vi "Dashboard Main.vi"() -> ()   [LabVIEW 2013]
uses:
  <vilib>/event_ctls.llb/eventvkey.ctl
  <vilib>/Rock Robotics/WPI/Dashboard/WPI_DashboardLogging Global.vi
  <vilib>/Utility/config.llb/Write Key (String).vi
  <vilib>/Utility/config.llb/Write Key (I32).vi
  KariFramework/CheckImageDistance.vi
  <vilib>/Utility/config.llb/NI_LVConfig.lvlib
panel:
  in  "Enable Vision":bool=TRUE
  out "Image Message":string="Timeout in Camera Communications"
  in  "Rec Mode":enum32{"Stop", "Record", "Playback"}(radio)
  in  "Dashboard Tab":T1(tab)=enum."Auto"
  out "Gear":bool
  in  "AccelRate":dbl=2.5
  out "Distance":dbl
  out "RPM":dbl
  out "Error":bool
  out "Right Motor":dbl(slide) scale=-1.0..1.0 scale format="%#.6g"
  out "StraightDrive":bool
  out "HalfDrive":bool
  out "Left Motor":dbl(slide) scale=-1.0..1.0
  in  "Camera Settings":T2={"Frame Rate"=30, "Compression"=30, "Size"=1} {"Frame Rate" scale=1.0..30.0; "Size" items=["640x480", "320x240", "160x120"]}
  out "MotorSliders R":cluster{"MotorSlide1":dbl, "MotorSlide2":dbl} {"MotorSlide2" scale=-1.0..1.0 scale format="%#_2e"; "MotorSlide1" scale=-1.0..1.0 scale format="%#_2e"}
  out "MotorChart R":cluster{"Numeric":dbl, "Numeric":dbl}(graph)
  out "MotorSliders L":T3 {"MotorSlide4 2" scale=0.0..14.0 scale format="%#_2e"; "MotorSlide2" scale=-1.0..1.0 scale format="%#_2e"; "MotorSlide1" scale=-1.0..1.0 scale format="%#_2e"}
  out "MotorChart L":T4(graph)
  out "Mode":T5(ring)=enum."Auto Disabled"
  out "Camera IP":string
  in  "DB Camera Config":bool
  out "fps":dbl format="%#.1g"
  out "Mbps":dbl format="%#.1g"
  out "Mbps 2":bool
  in  "DesiredAngle":dbl step=11.25
  out "Angle":dbl
  in  "AccelScale":dbl=1.0 step=1.0
  in  "% Cutoff":dbl=0.5
  out "NumHot":i32
  out "NumProcessed":i32
  in  "NumSamples":i32=5
  out "ProcessImage?":bool
  in  "Finished?":bool
  in  "Hot?":bool
  in  "Score cutoff":dbl=0.5
  in  "Color System":u16(ring)=2 items=["RGB", "HSL", "HSV", "HSI"]
  out "Distance (ft)":dbl
  in  "Color Components":T6={"Hue"={112.0, 144.0}, "Sat"={202.0, 255.0}, "Val"={237.0, 255.0}} {"Val" scale=0.0..255.0; "Sat" scale=0.0..255.0; "Hue" scale=0.0..255.0 scale format="%#_3g"}
  out "LoopTime":u32
  in  "Reset?":bool
  in  "Test Slider":dbl(slide) scale=0.0..100.0 scale format="%#_3g"
  in  "On/Off":bool caption="Solenoid"
  in  "Test Name":u16(ring) items=["Select the test to run...", "Example Test", "-------------------------------", "List of tests is built in robot code.", "Replace with your own automated tests."]
  in  "Test Tree":string(tree)
  in  "Motor":cluster{"Value":dbl, "Enable":bool} {"Value" scale=-1.0..1.0 scale format="%#_3g"}
  out "Progress":T7 {"Test Progress" scale=0.0..100.0}
  in  "Rev/Fwd":cluster{"Forward":bool, "Reverse":bool}
  in  "Test Ring":u16(ring) items=["Auto", "Fixed indoor", "Fixed outdoor 1", "Fixed outdoor 2", "Fixed fluorescent 1", "Fixed fluorescent 2", "Hold current"]
  in  "Listbox":i32(listbox)
  out "Tree":string(tree)
  out "Errors":T8(array[cluster])
  in  "Reset":bool
  out "Camera Image":T9(plugin-control)
  # "Left"
  # "Front"
  # "Right"
  # "Battery"
  # "Customize by placing controls and indicators here and name to\nmatch Dashboard Variables on robot."
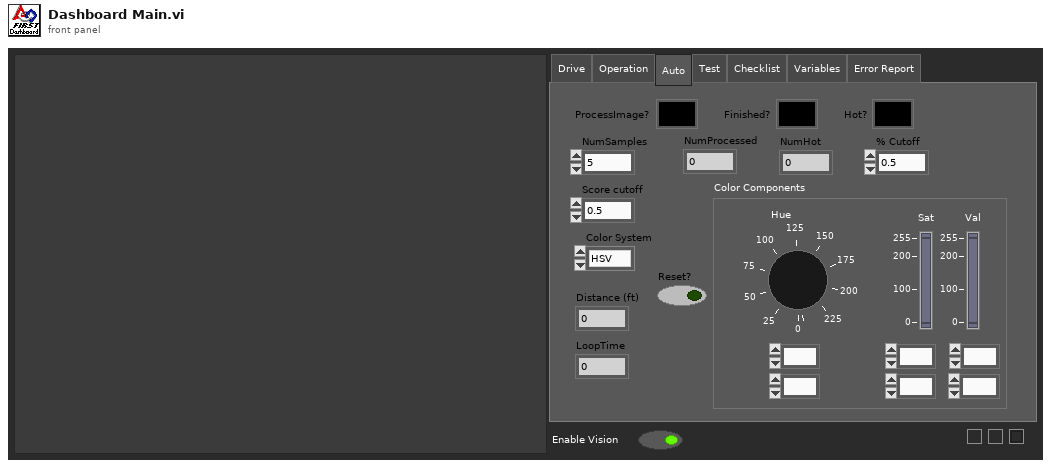
[diagram p1: front panel]
types:
  T1 = enum32{"Drive", "Operation", "Auto", "Test", "Checklist", "Variables", "Error Report"}
  T2 = cluster{"Frame Rate":i32, "Compression":i32, "Size":u16}
  T3 = cluster{"MotorSlide1":dbl, "MotorSlide2":dbl, "MotorSlide4 2":dbl}
  T4 = cluster{"Numeric":dbl, "Numeric":dbl, "Battery":sgl}
  T5 = enum8{"Tele-Op Disabled", "Tele-Op Enabled", "Auto Disabled", "Auto Enabled", "Test Disabled", "Test Enabled", ""}
  T6 = cluster{"Hue":cluster{dbl, dbl}, "Sat":cluster{dbl, dbl}, "Val":cluster{dbl, dbl}}
  T7 = cluster{"Test Progress":u8, "Test Progress Text":string}
  T8 = cluster{"status":bool, "code":i32, "location":string, "source":string}[]
  T9 = typedef "IMAQ Image.ctl" = refnum<image>
  T10 = enum32{"Drive", "Operation", "Auto", "Test", "Checklist", "Variables"}
  T11 = typedef "Image Type" = u32
  T12 = cluster{"Digital Inputs":bool[], "Digital Outputs":bool[]}
  T13 = cluster{"Competition mode":bool, "Robot Link":bool, "Autonomous":bool, "Enabled":bool, "E-Stop":bool, "Simulated":bool, "TestMode":bool, "Docked Window":bool}
  T14 = cluster{"Boolean":bool, "Numeric":i32, "String":string, "String":string}[]
  T15 = typedef "NI_LVConfig.lvlib/Config Data RefNum.ctl" = refnum<k1>
  T16 = typedef "eventvkey.ctl" = enum16{"ASCII", "Enter", "Return", "Shift", "Ctrl", "Alt", "Cmd", "Opt", "Caps", "NumLock", "Clear", "Break", "Up", "Down", "Left", "Right", "Insert", "Delete", "Home", "End", "PageUp", "PageDown", "Escape", "Help", "Pause", "ScrollLock", "F1", "F2", "F3", "F4", "F5", "F6", "F7", "F8", "F9", "F10", "F11", "F12", "F13", "F14", "F15", "F16", "F17", "F18", "F19", "F20", "F21", "F22", "F23", "F24", "Play", "VolumeUp", "VolumeDown", "Mute", "Two Byte Char"}
  T17 = cluster{"Image Size":bool, "Image Type":bool, "Pixel Value":bool, "ROI Information":bool, "Zoom Factor":bool}
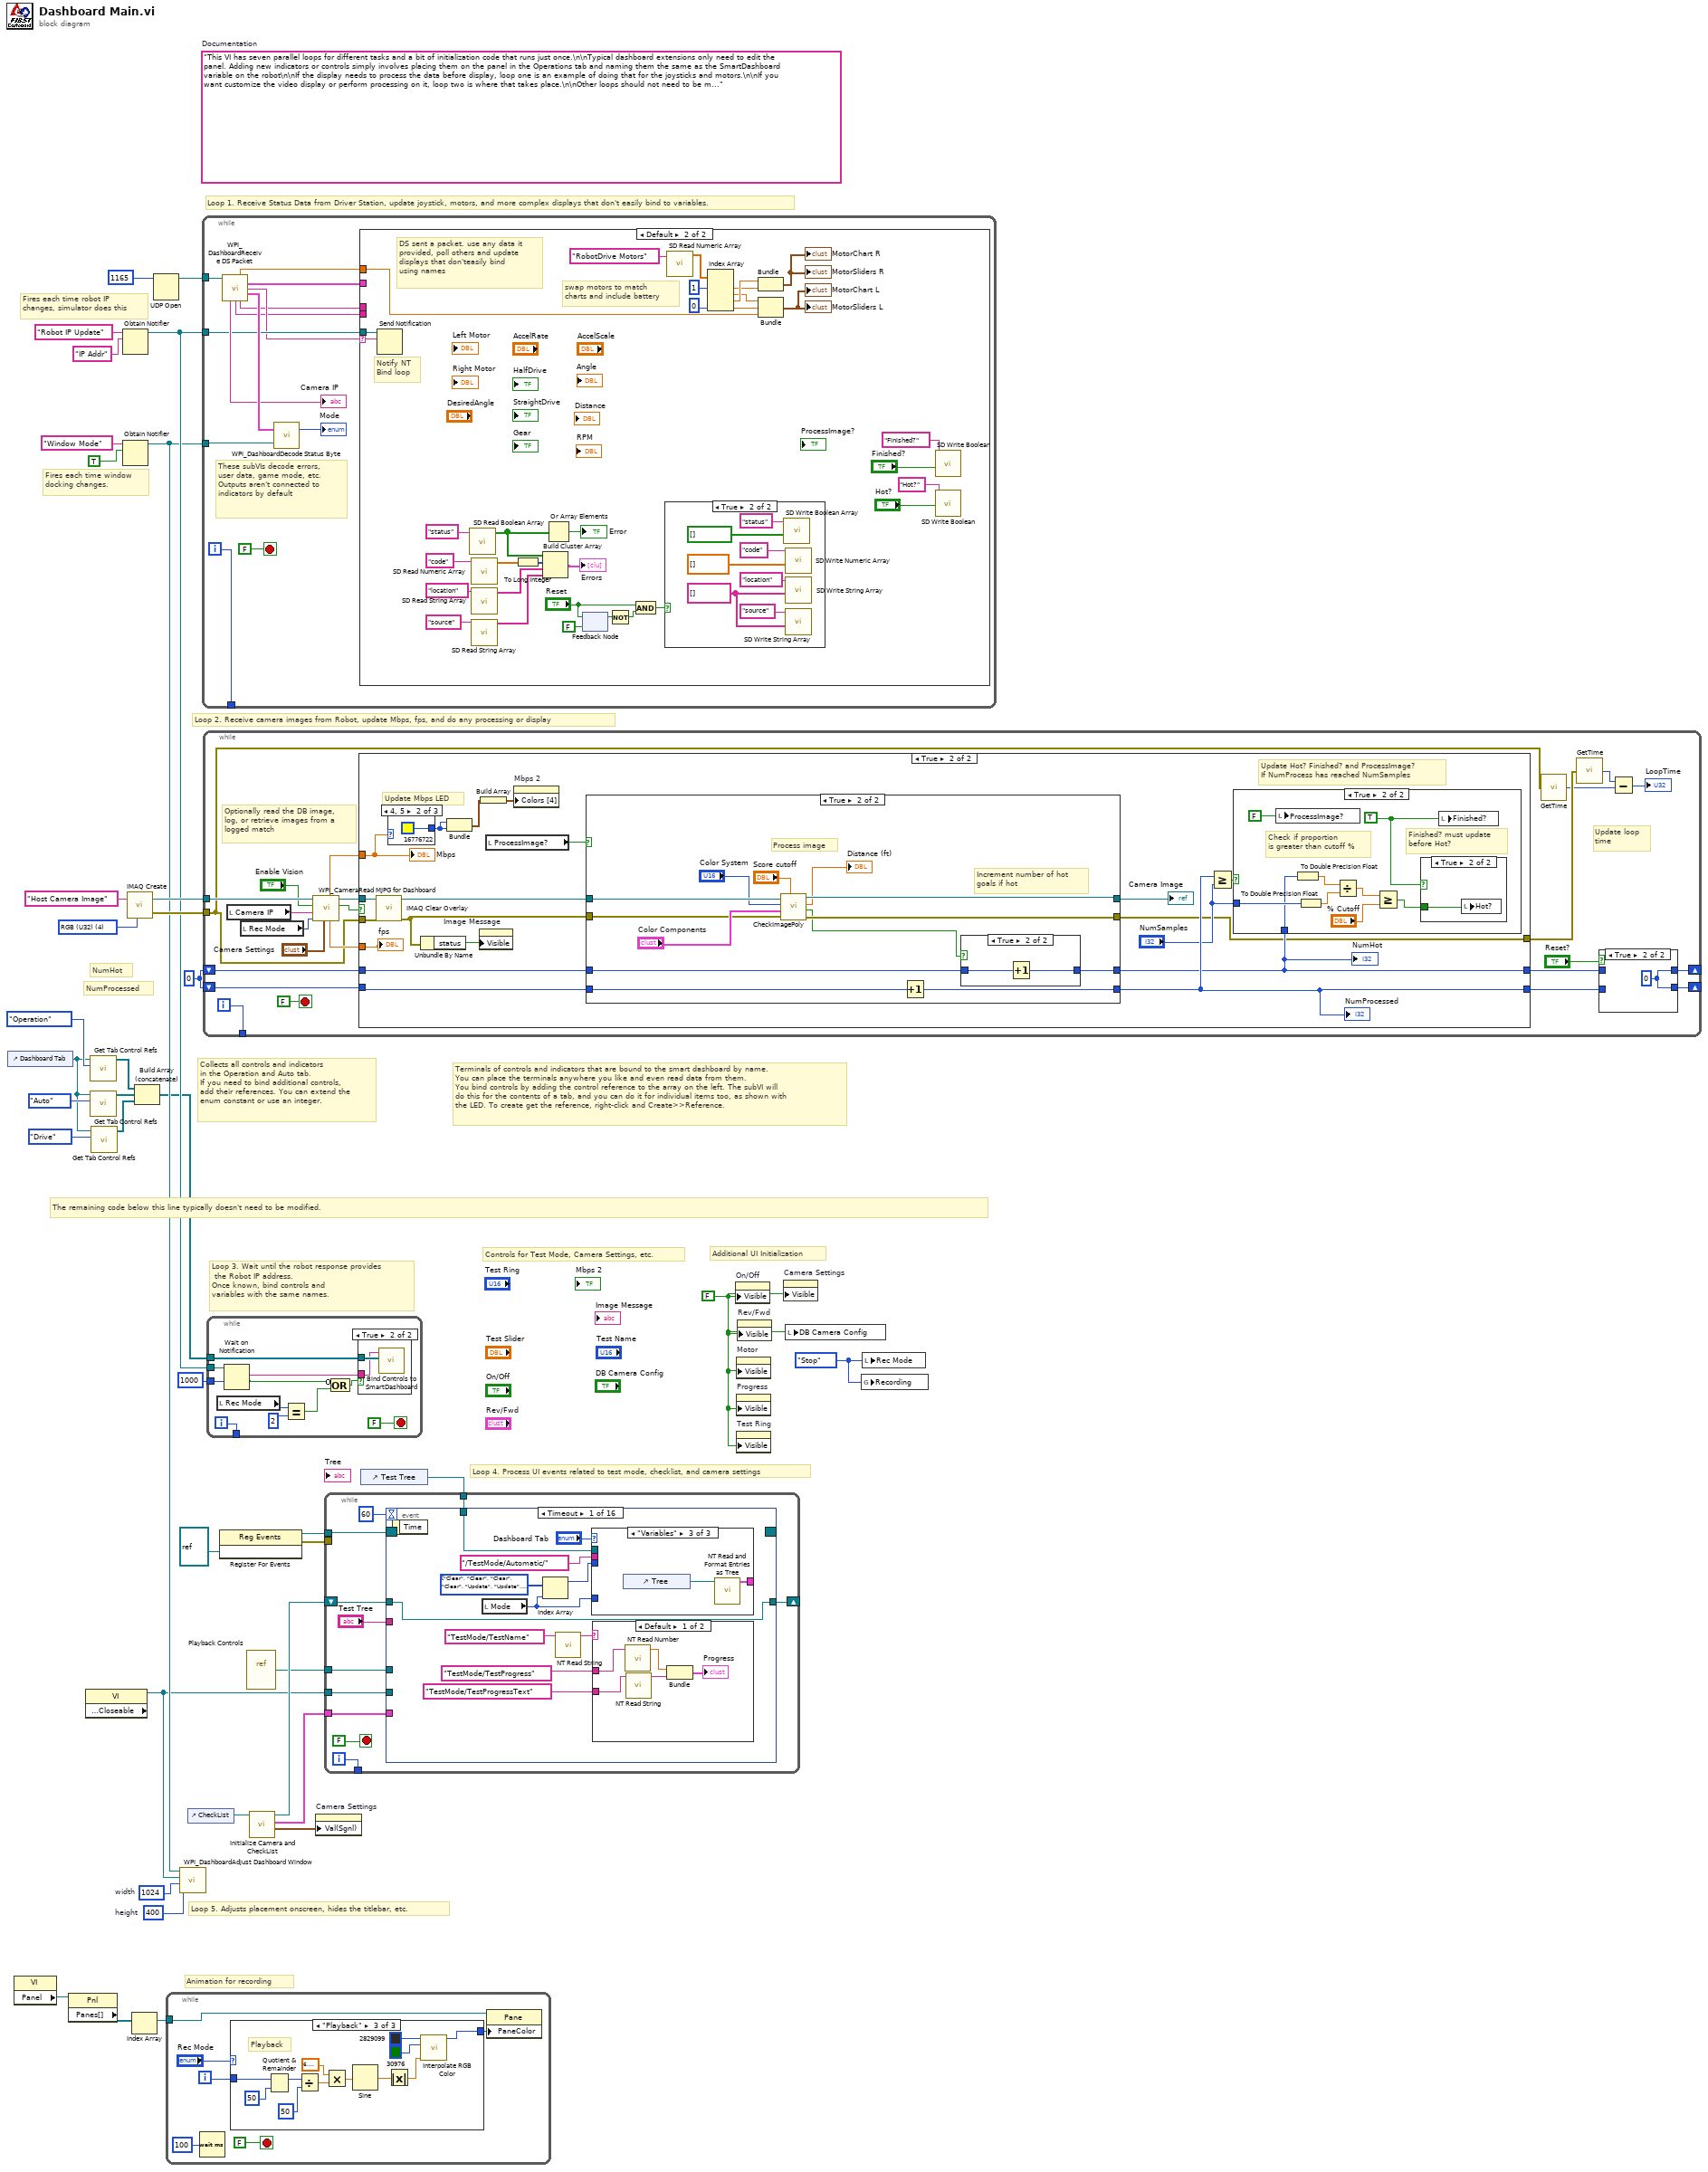
[diagram p0: block diagram]
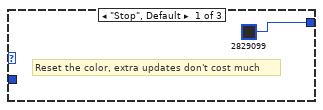
[diagram p2: hidden frame]
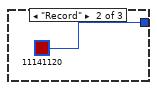
[diagram p3: hidden frame]
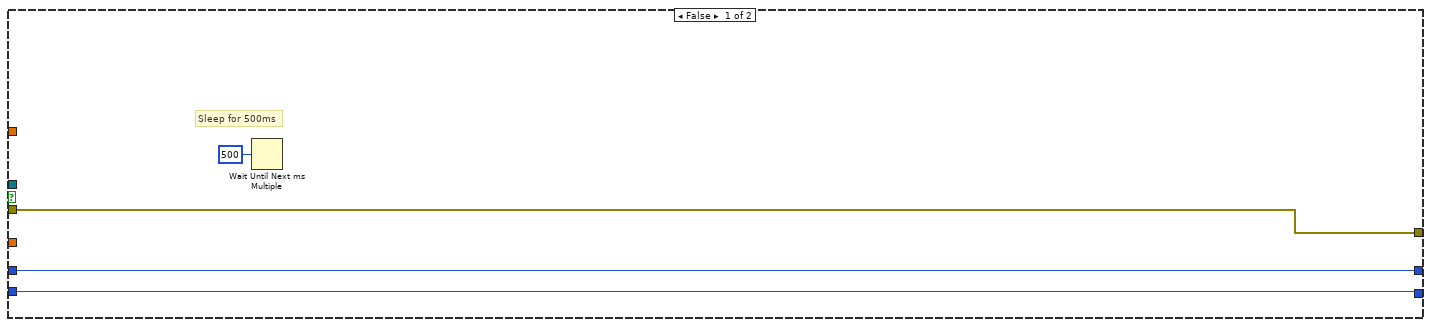
[diagram p6: hidden frame]
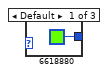
[diagram p11: hidden frame]
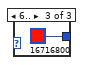
[diagram p12: hidden frame]
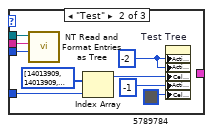
[diagram p14: hidden frame]
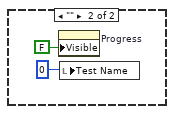
[diagram p15: hidden frame]
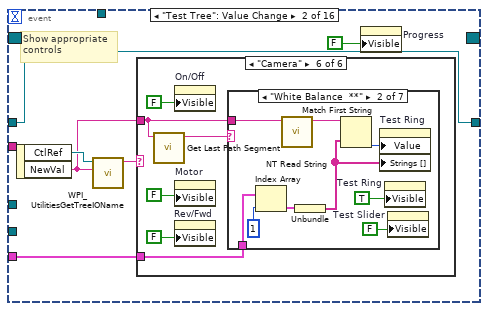
[diagram p16: hidden frame]
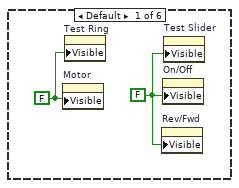
[diagram p17: hidden frame]
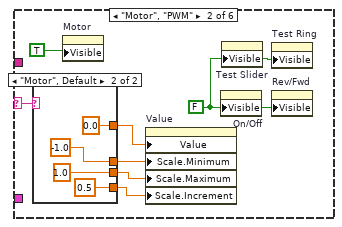
[diagram p18: hidden frame]
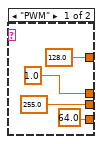
[diagram p19: hidden frame]
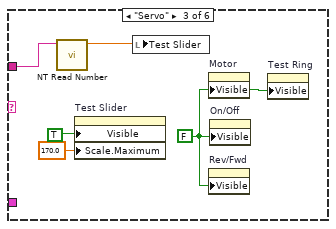
[diagram p20: hidden frame]
diagram:
  w1 = 0
  w10 = enum32{"Stop", "Record", "Playback"}."Stop" ("Rec Mode")
  w13 = 400  # height
  w14 = 1024  # width
  w27 = FALSE ("Visible")
  (unwired) "This VI has seven parallel loops for different tasks and a bit of initialization code that runs just once.\n\nTypical dashboard extensions only need to edit the panel. Adding new indicators or controls simply involves placing them on the panel in the Operations tab and naming them the same as the SmartDashboard variable on the robot\n\nIf the display needs to process the data before display, loop one is an example of doing that for the joysticks and motors.\n\nIf you want customize the video display or perform processing on it, loop two is where that takes place.\n\nOther loops should not need to be modified. They are pretty standard, and document the task they perform."  # Documentation
  w37 = T11 4 items=["Grayscale (U8)", "Grayscale (I16)", "Grayscale (SGL)", "Complex (CSG)", "RGB (U32)", "HSL (U32)", "RGB (U64)"] ("Image Type")
  # "NumProcessed"
  # "NumHot"
  # "Controls for Test Mode, Camera Settings, etc."
  # "Additional UI Initialization"
  # "Animation for recording"
  # "Fires each time robot IP\nchanges, simulator does this"
  # "Fires each time window\ndocking changes."
  # "Collects all controls and indicators\nin the Operation and Auto tab.\nIf you need to bind additional controls,\nadd their references. You can extend the\nenum constant or use an integer."
  # "The remaining code below this line typically doesn't need to be modified."
  # "Loop 4. Process UI events related to test mode, checklist, and camera settings"
  # "Terminals of controls and indicators that are bound to the smart dashboard by name.\nYou can place the terminals anywhere you like and even read data from them.\nYou bind controls by adding the control reference to the array on the left. The subVI will\ndo this for the contents of a tab, and you can do it for individual items too, as shown with\nthe LED. To create get the reference, right-click and Create>>Reference."
  # "Loop 3. Wait until the robot response provides\n the Robot IP address.\nOnce known, bind controls and\nvariables with the same names."
  # "Loop 5. Adjusts placement onscreen, hides the titlebar, etc."
  # "Loop 1. Receive Status Data from Driver Station, update joystick, motors, and more complex displays that don't easily bind to variables."
  # "Loop 2. Receive camera images from Robot, update Mbps, fps, and do any processing or display"
  n1 = control-ref of="Dashboard Tab"() -> (w3:refnum<vi>)
  n2 = property class="VI"() -> ("Panel"=w21:refnum<vi>)  [unwired: 2 in, 2 out]
  n3 = property class="Pnl"(reference=w21) -> ("Panes[]"=w22:refnum<vi>[])  [unwired: 1 in, 2 out]
  n4 = property class="VI" props=["Front Panel.Closeable"]() -> (reference out=w9:refnum<vi>)  [unwired: 2 in, 2 out]
  n5 = call <vilib>:"Get Tab Control Refs.vi"("Page Index"=T10."Operation" ("Dashboard Tab"), "TabControl in"=w3) -> ("ControlsOnPage"=w7:refnum<vi>[])  [unwired: 9 in]
  n6 = call <vilib>:"Get Tab Control Refs.vi"("Page Index"=T10."Auto" ("Dashboard Tab"), "TabControl in"=w3) -> ("ControlsOnPage"=w8:refnum<vi>[])  [unwired: 9 in]
  n7 = call <vilib>:"Get Tab Control Refs.vi"("Page Index"=T10."Drive" ("Dashboard Tab"), "TabControl in"=w3) -> ("ControlsOnPage"=w2:refnum<vi>[])  [unwired: 9 in]
  n8 = Obtain Notifier(name (unnamed)="Robot IP Update", notification data type="IP Addr" ("name (unnamed)")) -> (notifier out=w31:refnum<notifier>)  [unwired: 2 in, 2 out]
  n9 = Obtain Notifier(name (unnamed)="Window Mode", notification data type=TRUE) -> (notifier out=w12:refnum<notifier>)  [unwired: 2 in, 2 out]
  n10 = call "IMAQ Create"("Image Name"="Host Camera Image", "Image Type"=w37) -> ("New Image"=w35:T9, "error out"=w34:errorcluster)  [unwired: 2 in, 1 out]
  n11 = Index Array(array=w22) -> (element=w20:refnum<vi>)  [unwired: 1 in]
  n12 = Build Array (concatenate)(w7, w8, w2) -> (w6:refnum<vi>[])
  n13 = UDP Open(11:u16 1165 ("port")) -> (port=w38:refnum<k16>)  [unwired: 2 in, 4 out]
  n14 = while {
    tunnel: w20 -> [w41]
    i -> [w44]
    stop <- FALSE stop-if-true
    n15 = Wait (ms)(milliseconds to wait=u32 100) -> ()  [unwired: 1 out]
    n16 = case shown="\"Playback\"" "Rec Mode" {
      tunnel: w44 -> [_ _ w59]
      tunnel: [u32 2829099 ("Base Color") u32 11141120 ("Target Color") w48] -> w40
      frame "Stop", Default {
        # "Reset the color, extra updates don't cost much"
      }
      frame "Record" {
      }
      frame "Playback" {
        # "Playback"
        n17 = Quotient & Remainder(x=w59, y=u32 50 ("milliseconds to wait")) -> (x-y*floor(x/y)=w55:u32)  [unwired: 1 out]
        n18 = Divide(x=w55, y=u32 50 ("milliseconds to wait")) -> (x/y=w52:dbl)
        n19 = Multiply(x=6.283185307179586, y=w52) -> (x*y=w57:dbl)
        n20 = Sine(x=w57) -> (sin(x)=w56:dbl)
        n21 = Absolute Value(x=w56) -> (abs(x)=w49:dbl)
        n22 = call "Interpolate RGB Color.vi"("Proportion"=w49, "Target Color"=u32 30976, "Base Color"=u32 2829099) -> ("Result Color"=w48:u32)  [unwired: 8 in]
      }
    }
    n23 = property class="Pane"(reference=w41, "PaneColor"=w40) -> ()  [unwired: 1 in, 2 out]
  }
  n24 = call <vilib>:"WPI_DashboardAdjust Dashboard Window.vi"("height"=w13, "width"=w14, "reference in"=w9, "Notifier in"=w12) -> ()  [unwired: 8 in]
  n25 = control-ref of="CheckList"() -> (w11:refnum<vi>)
  n26 = while {
    tunnel: w38 -> [w70]
    tunnel: w31 -> [w65]
    tunnel: w12 -> [w69]
    tunnel: [w66] -> _
    i -> [w66]
    stop <- FALSE stop-if-true
    # "These subVIs decode errors, user data, game mode, etc.\nOutputs aren't connected to indicators by default"
    n27 = call <vilib>:"WPI_DashboardReceive DS Packet.vi"("Recv Socket"=w70) -> ("Battery"=w60:sgl, "Driver Station"=w61:T12, "Robot IP Address"=w64:string, "Status"=w71:T13, "Camera IP Address"=→"Camera IP":string, "Low Priority User Data"=w63:string, "High Priority User Data"=w62:string)  [unwired: 1 in, 7 out]
    n28 = call <vilib>:"WPI_DashboardDecode Status Byte.vi"("Window Mode Notifier"=w69, "Status"=w71) -> ("Mode"=→"Mode":T5)  [unwired: 1 out]
    n29 = case shown="Default" w64 {
      selector: w64 -> [_ w103]
      tunnel: w65 -> [_ w104]
      tunnel: w63 -> [_ _]
      tunnel: w62 -> [_ _]
      tunnel: w61 -> [_ _]
      tunnel: w60 -> [_ w102]
      frame "0.0.0.0" {
        # "DS not sending packets, or no robot exists yet.\nDon't poll the variables"
      }
      frame Default {
        # "Notify NT\nBind loop"
        # "DS sent a packet. use any data it\nprovided, poll others and update\ndisplays that don'teasily bind\nusing names"
        # "swap motors to match\ncharts and include battery"
        n30 = Send Notification(notification=w103, notifier=w104) -> ()  [unwired: 1 in, 2 out]
        n31 = call <vilib>:"SD Read Boolean Array.vi"("Name"="status") -> ("Boolean Array"=w82:bool[])  [unwired: 8 in, 2 out]
        n32 = call <vilib>:"SD Read Numeric Array.vi"("Name"="code") -> ("Numeric Array"=w81:dbl[])  [unwired: 8 in, 2 out]
        n33 = call <vilib>:"SD Read String Array.vi"("Name"="location") -> ("String Array"=w80:string[])  [unwired: 9 in, 1 out]
        n34 = call <vilib>:"SD Read String Array.vi"("Name"="source") -> ("String Array"=w79:string[])  [unwired: 9 in, 1 out]
        n35 = To Long Integer(number=w81) -> (32bit integer=w87:i32[])
        n36 = Build Cluster Array(w82, w87, w80, w79) -> (→"Errors":T14)
        n37 = Or Array Elements(Boolean array=w82) -> (logical OR=→"Error":bool)
        n38 = feedback #1(FALSE ("Reset")) -> (w90:bool)
        n39 = feedback-in #1("Reset") -> ()
        n40 = Not(x=w90) -> (.not. x?=w89:bool)
        n41 = And(x="Reset", y=w89) -> (x .and. y?=w88:bool)
        n42 = case shown="True" w88 {
          frame False {
          }
          frame True {
            w106 = string[] [] ("String Array")
            n43 = call <vilib>:"SD Write Boolean Array.vi"("Boolean Array"=bool[] [], "Name"="status") -> ()  [unwired: 8 in, 2 out]
            n44 = call <vilib>:"SD Write Numeric Array.vi"("Numeric Array"=dbl[] [], "Name"="code") -> ()  [unwired: 8 in, 2 out]
            n45 = call <vilib>:"SD Write String Array.vi"("String Array"=w106, "Name"="location") -> ()  [unwired: 8 in, 2 out]
            n46 = call <vilib>:"SD Write String Array.vi"("String Array"=w106, "Name"="source") -> ()  [unwired: 8 in, 2 out]
          }
        }
        n47 = call <vilib>:"SD Read Numeric Array.vi"("Name"="RobotDrive Motors") -> ("Numeric Array"=w101:dbl[])  [unwired: 8 in, 2 out]
        n48 = Index Array(array=w101, index #1=1, index #4=0) -> (element #1=w97:dbl, element #2=w96:dbl, element #3=w98:dbl, element #4=w93:dbl)  [unwired: 2 in]
        n49 = Bundle("Numeric"=w98, "Numeric"=w97) -> (→"MotorChart R" →"MotorSliders R":cluster{"Numeric":dbl, "Numeric":dbl})  [unwired: 1 in]
        n50 = Bundle("Numeric"=w96, "Numeric"=w93, "Battery"=w102) -> (→"MotorChart L" →"MotorSliders L":T4)  [unwired: 1 in]
        n51 = call <vilib>:"SD Write Boolean.vi"("Boolean"="Finished?", "Name"="Finished?") -> ()  [unwired: 8 in, 2 out]
        n52 = call <vilib>:"SD Write Boolean.vi"("Boolean"="Hot?", "Name"="Hot?") -> ()  [unwired: 8 in, 2 out]
      }
    }
  }
  n53 = while {
    tunnel: w35 -> [w133]
    tunnel: w34 -> [w118]
    tunnel: [w134] -> _
    shift-right: [w115] -> _
    shift-left: w1 -> [w123]
    shift-right: [w116] -> _
    shift-left: w1 -> [w124]
    i -> [w134]
    stop <- FALSE stop-if-true
    # "Update loop\ntime"
    # "Optionally read the DB image,\nlog, or retrieve images from a\nlogged match"
    n54 = local read "Camera IP"() -> (w126:string)
    n55 = local read "Rec Mode"() -> (w125:enum32{"Stop", "Record", "Playback"})
    n56 = call <vilib>:"WPI_CameraRead MJPG for Dashboard.vi"("Camera Settings"="Camera Settings", "Rec Mode"=w125, "Camera IP"=w126, "Enable"="Enable Vision", "Refnum in"=w133) -> ("Active"=w130:bool, "Refnum out"=w132:T9, "FPS"=w129:dbl, "Bandwidth (Mbps)"=w128:dbl)  [unwired: 3 in]
    n57 = case shown="True" w130 {
      tunnel: w132 -> [_ w157]
      tunnel: w128 -> [_ w156]
      tunnel: w129 -> [_ w155]
      tunnel: w124 -> [w140 w152]
      tunnel: w123 -> [w141 w151]
      tunnel: [w141 w148] -> w113
      tunnel: [w140 w147] -> w114
      tunnel: [w139 w145] -> w121
      tunnel: w118 -> [w139 w144]
      frame False {
        # "Sleep for 500ms"
        n58 = Wait Until Next ms Multiple(millisecond multiple=u32 500) -> ()  [unwired: 1 out]
      }
      frame True {
        # "Update Hot? Finished? and ProcessImage?\nIf NumProcess has reached NumSamples"
        # "Update Mbps LED"
        n59 = call "IMAQ Clear Overlay"("error in (no error)"=w144, "Image"=w157) -> ("error out"=w150:errorcluster, "Image Out"=w154:T9)  [unwired: 1 in, 7 out]
        n60 = case shown="4, 5" w156 {
          tunnel: [u32 6618880 ("Color Box") u32 16776722 ("Color Box") u32 16716800 ("Color Box")] -> w158
          frame Default {
          }
          frame 4, 5 {
          }
          frame 6.. {
          }
        }
        n61 = Unbundle By Name(w150) -> ("status"=w161:bool)
        n62 = Bundle("Color Box"=w158, "Color Box"=w158) -> (w160:cluster{"Color Box":u32, "Color Box":u32})  [unwired: 1 out]
        n63 = property on="Image Message" class="Str"("Visible"=w161) -> ()  [unwired: 2 in, 2 out]
        n64 = Build Array(w160) -> (w159:cluster{"Color Box":u32, "Color Box":u32}[])
        n65 = local read "ProcessImage?"() -> (w143:bool)
        n66 = property on="Mbps 2" class="Bool (strict)"("Colors [4]"=w159) -> ()  [unwired: 2 in, 2 out]
        n67 = case shown="True" w143 {
          tunnel: w154 -> [w175 w188]
          tunnel: [w175 w182] -> w153
          tunnel: w152 -> [w173 w179]
          tunnel: w151 -> [w174 w181]
          tunnel: w150 -> [w172 w184]
          tunnel: [w172 w183] -> w145
          tunnel: [w174 w180] -> w148
          tunnel: [w173 w178] -> w147
          frame False {
          }
          frame True {
            # "Process image"
            # "Increment number of hot\ngoals if hot"
            n68 = call-poly "CheckImagePoly.vi"("Score cutoff"="Score cutoff", "error in"=w184, "Color Components"="Color Components", "Color System"="Color System", "Image"=w188) -> ("error out"=w183:errorcluster, "Hot?"=w176:bool, "Distance (ft)"=→"Distance (ft)":dbl, "Image out"=w182:T9)  [unwired: 3 in]
            n69 = Increment(x=w181) -> (x+1=w180:i32)
            n70 = case shown="True" w176 {
              tunnel: w179 -> [w189 w191]
              tunnel: [w189 w190] -> w178
              frame False {
              }
              frame True {
                n71 = Increment(x=w191) -> (x+1=w190:i32)
              }
            }
          }
        }
        "Camera Image" <- w153
        "NumHot" <- w147
        "NumProcessed" <- w148
        n72 = Greater Or Equal?(x=w148, y="NumSamples") -> (x >= y?=w149:bool)
        n73 = case shown="True" w149 {
          tunnel: w147 -> [_ w169]
          tunnel: "NumSamples" -> [_ w170]
          frame False {
          }
          frame True {
            w162 = TRUE ("Finished?")
            # "Finished? must update\nbefore Hot?"
            # "Check if proportion\nis greater than cutoff %"
            n74 = local write "ProcessImage?"(FALSE ("ProcessImage?")) -> ()
            n75 = To Double Precision Float(number=w169) -> (double precision float=w167:dbl)
            n76 = To Double Precision Float(number=w170) -> (double precision float=w168:dbl)
            n77 = Divide(x=w167, y=w168) -> (x/y=w166:dbl)
            n78 = Greater Or Equal?(x=w166, y="% Cutoff") -> (x >= y?=w164:bool)
            n79 = case shown="True" w162 {
              tunnel: w164 -> [_ w171]
              frame False {
              }
              frame True {
                n80 = local write "Hot?"(w171) -> ()
              }
            }
            n81 = local write "Finished?"(w162) -> ()
          }
        }
        "Mbps" <- w156
        "fps" <- w155
      }
    }
    n82 = call "GetTime.vi"("error in"=w118) -> ("Time"=w120:u32)
    n83 = call "GetTime.vi"("error in"=w121) -> ("Time"=w122:u32)
    n84 = case shown="True" "Reset?" {
      tunnel: [w137 w138] -> w116
      tunnel: [w136 w138] -> w115
      tunnel: w114 -> [w137 _]
      tunnel: w113 -> [w136 _]
      frame False {
      }
      frame True {
        w138 = 0
      }
    }
    n85 = Subtract(x=w122, y=w120) -> (x-y=→"LoopTime":u32)
  }
  n86 = while {
    tunnel: w6 -> [w205]
    tunnel: w31 -> [w203]
    tunnel: [w201] -> _
    tunnel: u32 1000 ("milliseconds to wait") -> [w200]
    i -> [w201]
    stop <- FALSE stop-if-true
    n87 = local read "Rec Mode"() -> (w196:enum32{"Stop", "Record", "Playback"})
    n88 = Wait on Notification(notifier=w203, timeout in ms (-1)=w200) -> (notification=w202:string, timed out?=w198:bool)  [unwired: 2 in, 2 out]
    n89 = Equal?(x=w196, y=u16 2 ("Rec Mode")) -> (x = y?=w197:bool)
    n90 = Compound Arithmetic op=OR(invert w198, w197) -> (w199:bool)
    n91 = case shown="True" w199 {
      tunnel: w205 -> [_ w207]
      tunnel: w202 -> [_ w206]
      frame False {
      }
      frame True {
        n92 = call <vilib>:"Bind Controls to SmartDashboard.vi"("Bound Control Refs"=w207, "Server IP Address"=w206) -> ()  [unwired: 10 in]
      }
    }
  }
  n93 = register-events(refnum<vi> refnum) -> (reference out=w18:refnum<event-registration>, error out=w17:errorcluster)  [unwired: 2 in]
  n94 = vi-ref "Playback Controls.vi"() -> (w19:refnum<vi>)
  n95 = call "Initialize Camera and CheckList.vi"("ListBox in"=w11) -> ("Cluster"=w25:cluster{"value":i32, "value":i32, "index":i32}, "Array"=w26:cluster{string[]}[], "File Refnum"=w24:T15)  [unwired: 8 in]
  n96 = property on="Camera Settings" class="Clust (strict)"("Val(Sgnl)"=w25) -> ()  [unwired: 2 in, 2 out]
  n97 = control-ref of="Test Tree"() -> (w23:refnum<vi>)
  n98 = while {
    tunnel: w26 -> [w215]
    shift-right: [w214] -> _
    shift-left: w24 -> [w213]
    tunnel: [w212] -> _
    tunnel: w23 -> [w211]
    tunnel: w19 -> [w210]
    tunnel: w18 -> [w209]
    tunnel: w17 -> [_]
    tunnel: w9 -> [w208]
    i -> [w212]
    stop <- FALSE stop-if-true
    n99 = event shown="[0] Timeout" {
      selector: w209 -> [_ _ _ _ _ _ _ _ _ _ _ _ _ _ _ _]
      dyn-events: [_ _ _ _ _ _ _ _ _ _ _ _ _ w453 _ _] -> _
      timeout: u32 60 ("milliseconds to wait") -> [_ _ _ _ _ _ _ _ _ _ _ _ _ _ _ _]
      tunnel: w211 -> [w225 _ _ _ _ _ _ _ _ _ _ _ _ _ _ _]
      tunnel: "Test Tree" -> [_ _ _ _ _ _ _ _ w422 w430 w432 w436 w444 _ _ _]
      tunnel: w215 -> [_ w249 _ _ _ _ w386 w416 _ _ _ _ _ _ _ _]
      tunnel: [w219 w248 w347 w352 w360 w372 w385 w409 w421 w428 w431 w435 w443 w455 w469 w470] -> w214
      tunnel: w213 -> [w219 w248 w347 w352 w360 w372 w384 w409 w421 w428 w431 w435 w443 w455 w469 w470]
      tunnel: w210 -> [_ _ _ _ _ _ _ _ _ _ _ _ _ w456 _ w473]
      tunnel: w208 -> [_ _ _ _ _ _ _ _ _ _ _ _ _ w451 _ _]
      event Timeout {
        w224 = enum16{"Update", "Clear"}[] [enum."Clear", enum."Clear", enum."Clear", enum."Clear", enum."Update", enum."Update", enum."Clear"] items=["Update", "Clear"]
        n100 = event-data() -> ()  [unwired: 1 in, 1 out]
        n101 = local read "Mode"() -> (w222:T5)
        n102 = Index Array(array=w224, index=w222) -> (element=w223:enum16{"Update", "Clear"})
        n103 = call <vilib>:"NT Read String.vi"("Name"="TestMode/TestName") -> ("String"=w228:string)  [unwired: 9 in, 1 out]
        n104 = case shown="\"Variables\"" "Dashboard Tab" {
          tunnel: w225 -> [_ w238 _]
          tunnel: "/TestMode/Automatic/" ("Name Pattern") -> [_ w237 _]
          tunnel: w223 -> [_ w236 _]
          tunnel: w222 -> [_ w234 _]
          tunnel: [_ _ w240] -> _
          frame "Operation", Default {
          }
          frame "Test" {
            w233 = -2 ("Active Item:Row Number")
            n105 = call <vilib>:"NT Read and Format Entries as Tree.vi"("Operation"=w236, "Name Pattern"=w237, "Tree Refnum"=w238) -> ()  [unwired: 7 in, 2 out]
            n106 = Index Array(array=u32[] [14013909, 14013909, 14013909, 14013909, 14013909, 16777215, 14013909], index=w234) -> (element=w232:u32)
            n107 = property on="Test Tree" class="Tree (strict)"("Active Item Row Number"=w233, "ActiveColNum"=w233, "CellBG"=w232, "Active Item Row Number"=-1 ("Active Item:Row Number"), "CellBG"=u32 5789784 ("Color Box")) -> ()  [unwired: 2 in, 2 out]
          }
          frame "Variables" {
            n108 = control-ref of="Tree"() -> (w239:refnum<vi>)
            n109 = call <vilib>:"NT Read and Format Entries as Tree.vi"("Tree Refnum"=w239) -> ("Formatted Strings"=w240:cluster{"Name":string, "Value":string}[])  [unwired: 9 in, 1 out]
          }
        }
        n110 = case shown="Default" w228 {
          tunnel: "TestMode/TestProgress" ("Name") -> [w242 _]
          tunnel: "TestMode/TestProgressText" ("Name") -> [w241 _]
          frame Default {
            n111 = call <vilib>:"NT Read Number.vi"("Name"=w242) -> ("Numeric"=w243:dbl)  [unwired: 9 in, 1 out]
            n112 = call <vilib>:"NT Read String.vi"("Name"=w241) -> ("String"=w244:string)  [unwired: 9 in, 1 out]
            n113 = Bundle("Numeric"=w243, "String"=w244) -> (→"Progress":cluster{"Numeric":dbl, "String":string})  [unwired: 1 in]
          }
          frame "" {
            n114 = property on="Progress" class="Clust (strict)"("Visible"=FALSE) -> ()  [unwired: 2 in, 2 out]
            n115 = local write "Test Name"(u16 0) -> ()
          }
        }
      }
      event "Test Tree": Value Change {
        # "Show appropriate\ncontrols"
        n116 = event-data() -> ("CtlRef"=w252:refnum<vi>, "NewVal"=w250:string)  [unwired: 1 in]
        n117 = call <vilib>:"WPI_UtilitiesGetTreeIOName.vi"("NewVal"=w250, "TreeControl in"=w252) -> ("I/O Name"=w253:string)  [unwired: 9 in]
        n118 = case shown="\"Camera\"" w253 {
          selector: w253 -> [_ w260 _ w278 w287 _]
          tunnel: w250 -> [_ _ w275 w277 _ w294]
          tunnel: w249 -> [_ _ _ _ _ w293]
          frame Default {
            w255 = FALSE ("Visible")
            w254 = FALSE ("Visible")
            n119 = property on="Motor" class="Clust (strict)"("Visible"=w254) -> ()  [unwired: 2 in, 2 out]
            n120 = property on="Test Ring" class="Ring (strict)"("Visible"=w254) -> ()  [unwired: 2 in, 2 out]
            n121 = property on="Rev/Fwd" class="Clust (strict)"("Visible"=w255) -> ()  [unwired: 2 in, 2 out]
            n122 = property on="On/Off" class="Bool (strict)"("Visible"=w255) -> ()  [unwired: 2 in, 2 out]
            n123 = property on="Test Slider" class="Slide (strict)"("Visible"=w255) -> ()  [unwired: 2 in, 2 out]
          }
          frame "Motor", "PWM" {
            w261 = FALSE ("Visible")
            n124 = case shown="\"Motor\", Default" w260 {
              tunnel: [1.0 ("Value") -1.0 ("Value")] -> w259
              tunnel: [255.0 ("Value") 1.0 ("Value")] -> w258
              tunnel: [128.0 ("Value") 0.0 ("Value")] -> w257
              tunnel: [64.0 ("Value") 0.5 ("Value")] -> w256
              frame "PWM" {
              }
              frame "Motor", Default {
              }
            }
            n125 = property on="Motor" class="Clust (strict)"("Visible"=TRUE) -> ()  [unwired: 2 in, 2 out]
            n126 = property on="Value" class="Slide (strict)"("Value"=w257, "Scale.Minimum"=w259, "Scale.Maximum"=w258, "Scale.Increment"=w256) -> ()  [unwired: 2 in, 2 out]
            n127 = property on="On/Off" class="Bool (strict)"("Visible"=w261) -> ()  [unwired: 2 in, 2 out]
            n128 = property on="Test Slider" class="Slide (strict)"("Visible"=w261) -> ()  [unwired: 2 in, 2 out]
            n129 = property on="Test Ring" class="Ring (strict)"("Visible"=w261) -> ()  [unwired: 2 in, 2 out]
            n130 = property on="Rev/Fwd" class="Clust (strict)"("Visible"=w261) -> ()  [unwired: 2 in, 2 out]
          }
          frame "Servo" {
            w273 = FALSE ("Visible")
            n131 = call <vilib>:"NT Read Number.vi"("Name"=w275) -> ("Numeric"=w274:dbl)  [unwired: 9 in, 1 out]
            n132 = property on="Test Slider" class="Slide (strict)"("Visible"=TRUE, "Scale.Maximum"=170.0 ("Scale.Range:Maximum")) -> ()  [unwired: 2 in, 2 out]
            n133 = local write "Test Slider"(w274) -> ()
            n134 = property on="Motor" class="Clust (strict)"("Visible"=w273) -> ()  [unwired: 2 in, 2 out]
            n135 = property on="Rev/Fwd" class="Clust (strict)"("Visible"=w273) -> ()  [unwired: 2 in, 2 out]
            n136 = property on="On/Off" class="Bool (strict)"("Visible"=w273) -> ()  [unwired: 2 in, 2 out]
            n137 = property on="Test Ring" class="Ring (strict)"("Visible"=w273) -> ()  [unwired: 2 in, 2 out]
          }
          frame "Relay", "Solenoid" {
            w276 = FALSE ("Visible")
            n138 = property on="Motor" class="Clust (strict)"("Visible"=w276) -> ()  [unwired: 2 in, 2 out]
            n139 = property on="Test Slider" class="Slide (strict)"("Visible"=w276) -> ()  [unwired: 2 in, 2 out]
            n140 = Search and Replace String(input string=w277, search string="/Value  **", replace string="/Direction") -> (result string=w283:string)  [unwired: 5 in, 3 out]
            n141 = property on="Test Ring" class="Ring (strict)"("Visible"=w276) -> ()  [unwired: 2 in, 2 out]
            n142 = call <vilib>:"NT Read String.vi"("Name"=w283) -> ("String"=w281:string)  [unwired: 9 in, 1 out]
            n143 = Equal?(x="Both directions", y=w281) -> (x = y?=w279:bool)
            n144 = Not(x=w279) -> (.not. x?=w280:bool)
            n145 = property on="Rev/Fwd" class="Clust (strict)"("Visible"=w279) -> ()  [unwired: 2 in, 2 out]
            n146 = property on="On/Off" class="Bool (strict)"("Visible"=w280, "Caption.Text"=w278) -> ()  [unwired: 2 in, 2 out]
          }
          frame "Compressor", "Digital Out" {
            w286 = FALSE ("Visible")
            # "Get direction and finish"
            n147 = property on="Motor" class="Clust (strict)"("Visible"=w286) -> ()  [unwired: 2 in, 2 out]
            n148 = property on="Test Slider" class="Slide (strict)"("Visible"=w286) -> ()  [unwired: 2 in, 2 out]
            n149 = property on="Test Ring" class="Ring (strict)"("Visible"=w286) -> ()  [unwired: 2 in, 2 out]
            n150 = property on="On/Off" class="Bool (strict)"("Visible"=TRUE, "Caption.Text"=w287) -> ()  [unwired: 2 in, 2 out]
            n151 = property on="Rev/Fwd" class="Clust (strict)"("Visible"=FALSE) -> ()  [unwired: 2 in, 2 out]
          }
          frame "Camera" {
            n152 = call <vilib>:"Get Last Path Segment.vi"("String in"=w294) -> ("String out"=w295:string)  [unwired: 10 in]
            n153 = property on="On/Off" class="Bool (strict)"("Visible"=FALSE) -> ()  [unwired: 2 in, 2 out]
            n154 = property on="Motor" class="Clust (strict)"("Visible"=FALSE) -> ()  [unwired: 2 in, 2 out]
            n155 = property on="Rev/Fwd" class="Clust (strict)"("Visible"=FALSE) -> ()  [unwired: 2 in, 2 out]
            n156 = case shown="\"White Balance  **\"" w295 {
              tunnel: w294 -> [w301 w310 w319 w328 w337 _ w343]
              tunnel: w293 -> [w299 w307 w316 w325 w334 _ _]
              frame "Size  **" {
                n157 = Index Array(array=w299) -> (element=w298:cluster{string[]})  [unwired: 1 in]
                n158 = call <vilib>:"NT Read String.vi"("Name"=w301) -> ("String"=w300:string)  [unwired: 9 in, 1 out]
                n159 = Unbundle(w298) -> (w296:string[])
                n160 = Match First String(2:w296, 3:w300) -> (0:w297:i32)  [unwired: 1 out]
                n161 = property on="Test Ring" class="Ring (strict)"("Value"=w297, "Strings []"=w296) -> ()  [unwired: 2 in, 2 out]
                n162 = property on="Test Ring" class="Ring (strict)"("Visible"=TRUE) -> ()  [unwired: 2 in, 2 out]
                n163 = property on="Test Slider" class="Slide (strict)"("Visible"=FALSE) -> ()  [unwired: 2 in, 2 out]
              }
              frame "White Balance  **" {
                n164 = Index Array(array=w307, index=1) -> (element=w308:cluster{string[]})
                n165 = call <vilib>:"NT Read String.vi"("Name"=w310) -> ("String"=w309:string)  [unwired: 9 in, 1 out]
                n166 = Unbundle(w308) -> (w305:string[])
                n167 = Match First String(2:w305, 3:w309) -> (0:w304:i32)  [unwired: 1 out]
                n168 = property on="Test Ring" class="Ring (strict)"("Value"=w304, "Strings []"=w305) -> ()  [unwired: 2 in, 2 out]
                n169 = property on="Test Ring" class="Ring (strict)"("Visible"=TRUE) -> ()  [unwired: 2 in, 2 out]
                n170 = property on="Test Slider" class="Slide (strict)"("Visible"=FALSE) -> ()  [unwired: 2 in, 2 out]
              }
              frame "Exposure  **" {
                n171 = Index Array(array=w316, index=2) -> (element=w317:cluster{string[]})
                n172 = call <vilib>:"NT Read String.vi"("Name"=w319) -> ("String"=w318:string)  [unwired: 9 in, 1 out]
                n173 = Unbundle(w317) -> (w313:string[])
                n174 = Match First String(2:w313, 3:w318) -> (0:w314:i32)  [unwired: 1 out]
                n175 = property on="Test Ring" class="Ring (strict)"("Value"=w314, "Strings []"=w313) -> ()  [unwired: 2 in, 2 out]
                n176 = property on="Test Ring" class="Ring (strict)"("Visible"=TRUE) -> ()  [unwired: 2 in, 2 out]
                n177 = property on="Test Slider" class="Slide (strict)"("Visible"=FALSE) -> ()  [unwired: 2 in, 2 out]
              }
              frame "Exposure Priority  **" {
                n178 = Index Array(array=w325, index=3) -> (element=w326:cluster{string[]})
                n179 = call <vilib>:"NT Read String.vi"("Name"=w328) -> ("String"=w327:string)  [unwired: 9 in, 1 out]
                n180 = Unbundle(w326) -> (w322:string[])
                n181 = Match First String(2:w322, 3:w327) -> (0:w323:i32)  [unwired: 1 out]
                n182 = property on="Test Ring" class="Ring (strict)"("Value"=w323, "Strings []"=w322) -> ()  [unwired: 2 in, 2 out]
                n183 = property on="Test Ring" class="Ring (strict)"("Visible"=TRUE) -> ()  [unwired: 2 in, 2 out]
                n184 = property on="Test Slider" class="Slide (strict)"("Visible"=FALSE) -> ()  [unwired: 2 in, 2 out]
              }
              frame "Color Enable  **" {
                n185 = Index Array(array=w334, index=4) -> (element=w335:cluster{string[]})
                n186 = call <vilib>:"NT Read String.vi"("Name"=w337) -> ("String"=w336:string)  [unwired: 9 in, 1 out]
                n187 = Unbundle(w335) -> (w331:string[])
                n188 = Match First String(2:w331, 3:w336) -> (0:w332:i32)  [unwired: 1 out]
                n189 = property on="Test Ring" class="Ring (strict)"("Value"=w332, "Strings []"=w331) -> ()  [unwired: 2 in, 2 out]
                n190 = property on="Test Ring" class="Ring (strict)"("Visible"=TRUE) -> ()  [unwired: 2 in, 2 out]
                n191 = property on="Test Slider" class="Slide (strict)"("Visible"=FALSE) -> ()  [unwired: 2 in, 2 out]
              }
              frame Default {
                n192 = property on="Test Ring" class="Ring (strict)"("Visible"=FALSE) -> ()  [unwired: 2 in, 2 out]
                n193 = property on="Test Slider" class="Slide (strict)"("Visible"=FALSE) -> ()  [unwired: 2 in, 2 out]
              }
              frame "Brightness  **", "Color Level  **", "Compression  **", "FPS  **", "Sharpness  **" {
                n194 = call <vilib>:"NT Read Number.vi"("Name"=w343) -> ("Numeric"=w342:dbl)  [unwired: 9 in, 1 out]
                n195 = local write "Test Slider"(w342) -> ()
                n196 = property on="Test Slider" class="Slide (strict)"("Visible"=TRUE, "Scale.Maximum"=100.0 ("Scale.Range:Maximum")) -> ()  [unwired: 2 in, 2 out]
                n197 = property on="Test Ring" class="Ring (strict)"("Visible"=FALSE) -> ()  [unwired: 2 in, 2 out]
              }
            }
          }
        }
        n198 = property on="Progress" class="Clust (strict)"("Visible"=FALSE) -> ()  [unwired: 2 in, 2 out]
      }
      event "Test Name": Mouse Enter {
        # "Populate the ring with the list of tests"
        n199 = event-data() -> ()  [unwired: 1 in, 1 out]
        n200 = call <vilib>:"NT Read String Array.vi"("Name"="TestMode/TestList") -> ("String Array"=w351:string[])  [unwired: 9 in, 1 out]
        n201 = Build Array (concatenate)("Select the test to run...", w351) -> (w350:string[])
        n202 = property on="Test Name" class="Ring (strict)"("Strings []"=w350) -> ()  [unwired: 2 in, 2 out]
      }
      event "Test Name": Value Change {
        w353 = FALSE ("Visible")
        # "Tell the robot the test name to run"
        n203 = event-data() -> ("NewVal"=w357:u16)  [unwired: 1 in]
        n204 = property on="Test Name" class="Ring (strict)"() -> ("Strings []"=w358:string[])  [unwired: 2 in, 2 out]
        n205 = local write "Progress"(T7 {"Test Progress"=0, "Test Progress Text"=""} ("Progress")) -> ()
        n206 = Index Array(array=w358, index=w357) -> (element=w356:string)
        n207 = call <vilib>:"NT Write String.vi"("String"=w356, "Name"="TestMode/TestName") -> ()  [unwired: 9 in, 1 out]
        n208 = property on="Progress" class="Clust (strict)"("Visible"=TRUE) -> ()  [unwired: 2 in, 2 out]
        n209 = property on="Motor" class="Clust (strict)"("Visible"=w353) -> ()  [unwired: 2 in, 2 out]
        n210 = property on="Test Slider" class="Slide (strict)"("Visible"=w353) -> ()  [unwired: 2 in, 2 out]
        n211 = property on="On/Off" class="Bool (strict)"("Visible"=w353) -> ()  [unwired: 2 in, 2 out]
        n212 = property on="Rev/Fwd" class="Clust (strict)"("Visible"=w353) -> ()  [unwired: 2 in, 2 out]
        n213 = property on="Test Ring" class="Ring (strict)"("Visible"=w353) -> ()  [unwired: 2 in, 2 out]
      }
      event "Listbox": Double Click {
        n214 = event-data() -> ("PlatMods.Shift"=w361:bool, "Row"=w363:i32)  [unwired: 1 in]
        n215 = case shown="True" w361 {
          tunnel: w363 -> [w367 _]
          tunnel: 1 -> [w366 _]
          frame False {
            n216 = property on="Listbox" class="LstBox (strict)"() -> ("Item Symbols"=w365:i32[])  [unwired: 2 in, 2 out]
            n217 = Replace Array Subset(array=w365, new element=w366, index=w367) -> (w364:i32[])
            n218 = property on="Listbox" class="LstBox (strict)"("Item Symbols"=w364) -> ()  [unwired: 2 in, 2 out]
          }
          frame True {
            w368 = 0 ("Top Row")
            n219 = property on="Listbox" class="LstBox (strict)"() -> ("Number of Rows"=w370:u32)  [unwired: 2 in, 2 out]
            n220 = Initialize Array(0, w370) -> (w369:i32[])
            n221 = property on="Listbox" class="LstBox (strict)"("Top Row"=w368, "Value"=w368, "Item Symbols"=w369) -> ()  [unwired: 2 in, 2 out]
          }
        }
      }
      event "Listbox": Key Down {
        n222 = event-data() -> ("VKey"=w374:T16)  [unwired: 1 in]
        n223 = case shown="\"Left\", \"Right\"" w374 {
          selector: w374 -> [w379 _]
          tunnel: eventvkey."Left" ("VKey") -> [w377 _]
          frame "Left", "Right" {
            n224 = Equal?(x=w377, y=w379) -> (x = y?=w378:bool)
            n225 = Select(t=0, s=w378, f=1) -> (s? t:f=w380:i32)
            n226 = property on="Listbox" class="LstBox (strict)"() -> ("Item Symbols"=w383:i32[])  [unwired: 2 in, 2 out]
            n227 = Replace Array Subset(array=w383, new element=w380, index="Listbox") -> (w382:i32[])
            n228 = property on="Listbox" class="LstBox (strict)"("Item Symbols"=w382) -> ()  [unwired: 2 in, 2 out]
          }
          frame Default {
          }
        }
      }
      event "DB Camera Config": Value Change {
        n229 = event-data() -> ("NewVal"=w387:bool)  [unwired: 1 in]
        n230 = case shown="False" w387 {
          tunnel: w386 -> [w396 _]
          tunnel: [w389 w407] -> w385
          tunnel: w384 -> [w388 w407]
          frame False {
            w403 = "Camera"
            w406 = FALSE ("Visible")
            n231 = local read "Camera Settings"() -> (w395:T2)
            n232 = Index Array(array=w396) -> (element=w399:cluster{string[]})  [unwired: 1 in]
            n233 = Unbundle(w395) -> ("Frame Rate"=w394:i32, "Compression"=w393:i32, "Size"=w397:u16)
            n234 = Unbundle(w399) -> (w398:string[])
            n235 = Index Array(array=w398, index=w397) -> (element=w392:string)
            n236 = call-poly <vilib>:"Write Key.vi"("section"=w403, "value"=w392, "key"="Size", "refnum"=w388) -> ("refnum out"=w405:T15)  [unwired: 2 in, 5 out]
            n237 = call-poly <vilib>:"Write Key.vi"("section"=w403, "value"=w394, "key"="FrameRate", "refnum"=w405) -> ("refnum out"=w404:T15)  [unwired: 1 in, 6 out]
            n238 = property on="Camera Settings" class="Clust (strict)"("Visible"=w406) -> ()  [unwired: 2 in, 2 out]
            n239 = local write "DB Camera Config"(w406) -> ()
            n240 = call-poly <vilib>:"Write Key.vi"("section"=w403, "value"=w393, "key"="Compression", "refnum"=w404) -> ("refnum out"=w390:T15)  [unwired: 1 in, 6 out]
            n241 = call <vilib>:"Close Config Data.vi"("refnum"=w390) -> ("file path"=w391:path)  [unwired: 2 in, 8 out]
            n242 = call <vilib>:"Open Config Data.vi"("configuration file path"=w391) -> ("refnum"=w389:T15)  [unwired: 8 in, 2 out]
          }
          frame True {
            n243 = property on="Camera Settings" class="Clust (strict)"("Visible"=TRUE) -> ()  [unwired: 2 in, 2 out]
          }
        }
      }
      event "Camera Settings": Value Change {
        n244 = event-data() -> ("NewVal"=w420:T2)  [unwired: 1 in]
        n245 = Index Array(array=w416) -> (element=w415:cluster{string[]})  [unwired: 1 in]
        n246 = Unbundle(w420) -> ("Frame Rate"=w411:i32, "Compression"=w410:i32, "Size"=w413:u16)
        n247 = Unbundle(w415) -> (w414:string[])
        n248 = Index Array(array=w414, index=w413) -> (element=w412:string)
        n249 = Format Into String(format string="%s   %dfps   %d%%", w412, w411, w410) -> (resulting string=w417:string)  [unwired: 2 in, 1 out]
        n250 = Build Array(w417) -> (w418:string[])
        n251 = property on="DB Camera Config" class="Bool (strict)"("Strings [4]"=w418) -> ()  [unwired: 2 in, 2 out]
      }
      event "Motor.Enable": Value Change {
        n252 = event-data() -> ("NewVal"=w426:bool)  [unwired: 1 in]
        n253 = Unbundle("Motor") -> ("Value"=w425:dbl)  [unwired: 1 out]
        n254 = Select(t=w425, s=w426, f=0.0) -> (s? t:f=w423:dbl)
        n255 = call <vilib>:"NT Write Number.vi"("Numeric"=w423, "Name"=w422) -> ()  [unwired: 9 in, 1 out]
      }
      event "Test Slider": Value Change {
        n256 = event-data() -> ("NewVal"=w429:dbl)  [unwired: 1 in]
        n257 = call <vilib>:"NT Write Number.vi"("Numeric"=w429, "Name"=w430) -> ()  [unwired: 9 in, 1 out]
      }
      event "On/Off": Value Change {
        n258 = event-data() -> ("NewVal"=w434:bool)  [unwired: 1 in]
        n259 = Boolean To (0,1)(Boolean=w434) -> (0, 1=w433:i16)
        n260 = call <vilib>:"NT Write Number.vi"("Numeric"=w433, "Name"=w432) -> ()  [unwired: 9 in, 1 out]
      }
      event "Rev/Fwd": Value Change {
        n261 = event-data() -> ("NewVal.Forward"=w442:bool, "NewVal.Reverse"=w441:bool)  [unwired: 1 in]
        n262 = Boolean To (0,1)(Boolean=w442) -> (0, 1=w438:i16)
        n263 = Boolean To (0,1)(Boolean=w441) -> (0, 1=w440:i16)
        n264 = Negate(x=w440) -> (-x=w439:i16)
        n265 = Add(x=w438, y=w439) -> (x+y=w437:i16)
        n266 = call <vilib>:"NT Write Number.vi"("Numeric"=w437, "Name"=w436) -> ()  [unwired: 9 in, 1 out]
      }
      event "Test Ring": Value Change {
        n267 = event-data() -> ("NewVal"=w446:u16)  [unwired: 1 in]
        n268 = property on="Test Ring" class="Ring (strict)"() -> ("Strings []"=w447:string[])  [unwired: 2 in, 2 out]
        n269 = Index Array(array=w447, index=w446) -> (element=w445:string)
        n270 = call <vilib>:"NT Write String.vi"("String"=w445, "Name"=w444) -> ()  [unwired: 9 in, 1 out]
      }
      event "Rec Mode": Value Change {
        # "Update globals for recording mode and path to read log from.\nClear when logging and let NetworkTables set path for vision to\nuse."
        n271 = event-data() -> ("NewVal"=w457:enum32{"Stop", "Record", "Playback"})  [unwired: 1 in]
        n272 = global write "WPI_DashboardLogging Global.vi" "Logging Filename"(path "") -> ()
        n273 = case shown="\"Stop\", \"Record\"" w457 {
          tunnel: w456 -> [_ w459 w467]
          tunnel: [_ _ w466] -> w453
          tunnel: [_ _ w465] -> _
          tunnel: w451 -> [_ _ w463]
          tunnel: cluster{i32, i32} {-250, 170} -> [_ _ w462]
          tunnel: [_ _ T17 {"Image Size"=TRUE, "Image Type"=TRUE, "Pixel Value"=TRUE, "ROI Information"=TRUE, "Zoom Factor"=FALSE} ("Image Information Shown:All Elements")] -> w449
          tunnel: [_ _ TRUE ("Zoom Factor")] -> w448
          frame Default {
          }
          frame "Stop", "Record" {
            # "Place Window too"
            n274 = invoke class="VI" method="FP.Close"(reference=w459) -> (reference out=w458:refnum<vi>)  [unwired: 2 in, 2 out]
            n275 = invoke class="VI" method="Abort VI"(reference=w458) -> ()  [unwired: 2 in, 3 out]
          }
          frame "Playback" {
            n276 = call "Open Playback Panel.vi"("Offset"=w462, "DB VI Ref"=w463, "Playback in"=w467) -> ("Playback out"=w464:refnum<vi>)  [unwired: 8 in]
            n277 = register-events(w464) -> (reference out=w466:refnum<event-registration>, error out=w465:errorcluster)  [unwired: 2 in]
          }
        }
        n278 = global write "WPI_DashboardLogging Global.vi" "Recording"(w457) -> ()
        n279 = property on="Camera Image" class="ImageControl"("Image Information Shown"=w449, "Image Information Visible"=w448) -> ()  [unwired: 2 in, 2 out]
        n280 = call <vilib>:"WPI_DashboardNT Log FieldName Cache.vi"("Operation"=enum16{"Lookup/Add", "Index", "Clear"}."Clear") -> ()  [unwired: 8 in, 3 out]
      }
      event Panel Close {
        w468 = enum32{"Stop", "Record", "Playback"}."Stop" ("Rec Mode")
        n281 = event-data() -> ()  [unwired: 1 in, 4 out]
        n282 = local write "Rec Mode"(w468) -> ()
        n283 = global write "WPI_DashboardLogging Global.vi" "Recording"(w468) -> ()
      }
      event Panel Close {
        # "Abort playback window and ourself"
        n284 = event-data() -> ()  [unwired: 1 in, 4 out]
        n285 = invoke class="VI" method="FP.Close"(reference=w473) -> (reference out=w472:refnum<vi>)  [unwired: 2 in, 2 out]
        n286 = invoke class="VI" method="Abort VI"(reference=w472) -> (error out=w471:errorcluster)  [unwired: 2 in, 2 out]
        n287 = invoke class="VI" method="Abort VI"(error in=w471) -> ()  [unwired: 2 in, 3 out]
      }
    }
  }
  n288 = property on="On/Off" class="Bool (strict)"("Visible"=w27) -> ()  [unwired: 2 in, 2 out]
  n289 = property on="Motor" class="Clust (strict)"("Visible"=w27) -> ()  [unwired: 2 in, 2 out]
  n290 = property on="Progress" class="Clust (strict)"("Visible"=w27) -> ()  [unwired: 2 in, 2 out]
  n291 = property on="Test Ring" class="Ring (strict)"("Visible"=w27) -> ()  [unwired: 2 in, 2 out]
  n292 = property on="Rev/Fwd" class="Clust (strict)"("Visible"=w27) -> ()  [unwired: 2 in, 2 out]
  n293 = property on="Camera Settings" class="Clust (strict)"("Visible"=w27) -> ()  [unwired: 2 in, 2 out]
  n294 = local write "DB Camera Config"(w27) -> ()
  n295 = global write "WPI_DashboardLogging Global.vi" "Recording"(w10) -> ()
  n296 = local write "Rec Mode"(w10) -> ()
